vi "Initialize temp channel differential.vi"(6 "error in":errorcluster, 8 "Physical channel":tag) -> (0 "error out":errorcluster, 2 "task out":refnum<k21>)   [LabVIEW 2011]
uses:
  <vilib>/DAQmx/create/scale.llb/DAQmx Create Scale (Linear).vi
  <vilib>/DAQmx/create/channels.llb/DAQmx Create Channel (AI-Voltage-Basic).vi
  <vilib>/DAQmx/configure/timing.llb/DAQmx Timing (Sample Clock).vi
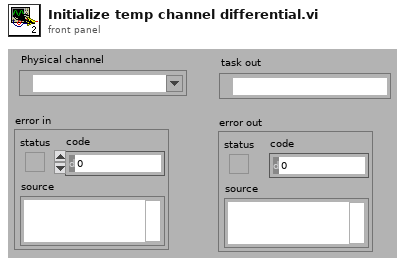
[diagram p1: front panel]
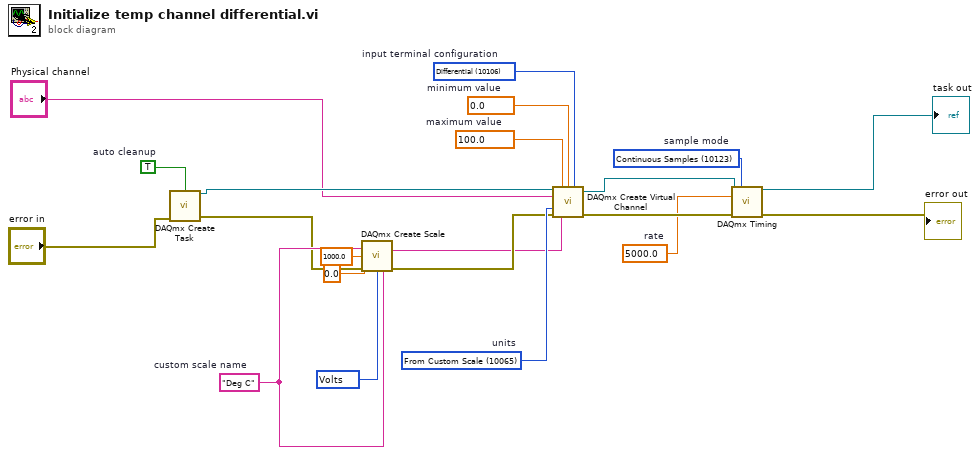
[diagram p0: block diagram]
diagram:
  w9 = 10348 items=["Volts"=10348, "Amps"=10342, "Deg F"=10144, "Deg C"=10143, "Deg R"=10145, "Kelvins"=10325, "Strain"=10299, "Ohms"=10384, "Hz"=10373, "Seconds"=10364, "Meters"=10219, "Inches"=10379, "Degrees"=10146, "Radians"=10273, "g"=10186, "m/s^2"=12470, "Pascals"=10081, "From TEDS"=12516] ("pre-scaled units")
  w6 = "Deg C"  # custom scale name
  w17 = 10123 items=["Finite Samples"=10178, "Continuous Samples"=10123, "Hardware Timed Single Point"=12522]  # sample mode
  w16 = 5000.0  # rate
  w15 = 10106 items=["default"=-1, "RSE"=10083, "NRSE"=10078, "Differential"=10106, "Pseudodifferential"=12529]  # input terminal configuration
  w14 = 10065 items=["Volts"=10348, "From Custom Scale"=10065]  # units
  w13 = 0.0  # minimum value
  w12 = 100.0  # maximum value
  w11 = TRUE  # auto cleanup
  n1 = call <vilib>:"DAQmx Create Task.vi"("auto cleanup"=w11, "error in"="error in") -> ("task out"=w3:refnum<k21>, "error out"=w5:errorcluster)  [unwired: 3 in, 9 out]
  n2 = call-poly <vilib>:"DAQmx Create Scale.vi"("name"=w6, "slope"=1000.0, "y-intercept"=0.0, "error in"=w5, "pre-scaled units"=w9, "scaled units"=w6) -> ("scale out"=w2:tag, "error out"=w4:errorcluster)  [unwired: 8 out]
  n3 = call-poly <vilib>:"DAQmx Create Virtual Channel.vi"("task in"=w3, "maximum value"=w12, "minimum value"=w13, "input terminal configuration"=w15, "physical channels"="Physical channel", "units"=w14, "error in"=w4, "custom scale name"=w2) -> ("task out"=w18:refnum<k21>, "error out"=w19:errorcluster)  [unwired: 1 in, 5 out]
  n4 = call-poly <vilib>:"DAQmx Timing.vi"("task/channels in"=w18, "sample mode"=w17, "rate"=w16, "error in"=w19) -> ("task out"=→"task out":refnum<k21>, "error out"=→"error out":errorcluster)  [unwired: 3 in, 7 out]
